vi "Segment_e.vi"(11 "Input in Binary":bool[](array[boolean])) -> (3 "Segment e":bool)   [LabVIEW 2024]
panel:
  out "D":bool
  out "C":bool
  out "B":bool
  out "A":bool
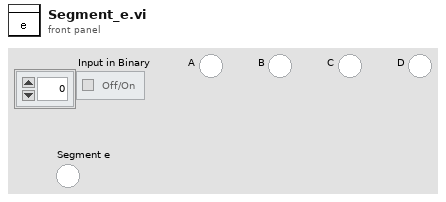
[diagram p1: front panel]
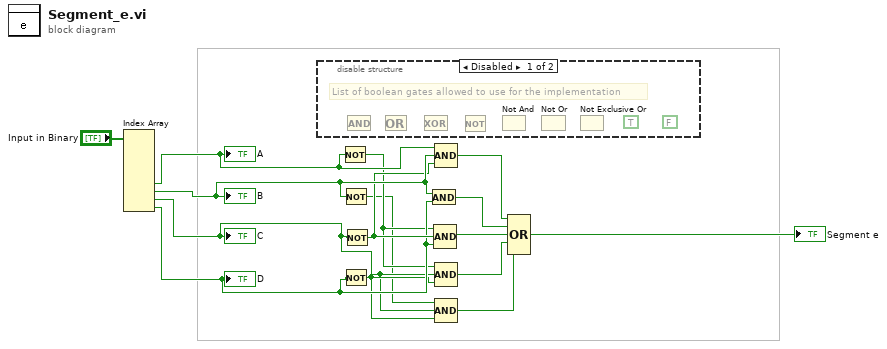
[diagram p0: block diagram]
diagram:
  n1 = Index Array(array="Input in Binary") -> (element #5=w14:bool, element #6=w13:bool, element #7=w3:bool, element #8=w11:bool)  [unwired: 8 in, 4 out]
  "A" <- w14
  "B" <- w13
  "C" <- w3
  "D" <- w11
  n2 = disable-structure shown="Disabled" {
    frame Disabled {
      (unwired) FALSE
      (unwired) TRUE
      # "List of boolean gates allowed to use for the implementation"
      n3 = And() -> ()  [unwired: 2 in, 1 out]
      n4 = Or() -> ()  [unwired: 2 in, 1 out]
      n5 = Exclusive Or() -> ()  [unwired: 2 in, 1 out]
      n6 = Not() -> ()  [unwired: 1 in, 1 out]
      n7 = Not And() -> ()  [unwired: 2 in, 1 out]
      n8 = Not Or() -> ()  [unwired: 2 in, 1 out]
      n9 = Not Exclusive Or() -> ()  [unwired: 2 in, 1 out]
    }
    frame Enabled {
    }
  }
  n10 = Not(x=w14) -> (.not. x?=w5:bool)
  n11 = Not(x=w13) -> (.not. x?=w2:bool)
  n12 = Not(x=w11) -> (.not. x?=w4:bool)
  n13 = Not(x=w3) -> (.not. x?=w12:bool)
  n14 = And(x=w13, y=w11) -> (x .and. y?=w9:bool)
  n15 = Compound Arithmetic op=AND(w5, w12, w11) -> (w8:bool)
  n16 = Compound Arithmetic op=AND(w14, w13, w12) -> (w10:bool)
  n17 = Compound Arithmetic op=AND(w5, w3, w4) -> (w7:bool)
  n18 = Compound Arithmetic op=AND(w2, w3, w4) -> (w6:bool)
  n19 = Compound Arithmetic op=OR(w10, w9, w8, w7, w6) -> (→"Segment e":bool)
